vi "Shallow Search Priv.vi"(0 "Tree Dictionary In":variant, 5 "Unique ID":string, 7 "Name":string, 11 "error in":errorcluster) -> (4 "Tree Dictionary Out":variant, 6 "IDs":string[](array[string]), 15 "error out":errorcluster)   [LabVIEW 2016, in "Tree Manager.lvclass"]
uses:
  Tree Manager.lvclass
  Typedefs/Tree.ctl
  <vilib>/Utility/error.llb/Error Cluster From Error Code.vi
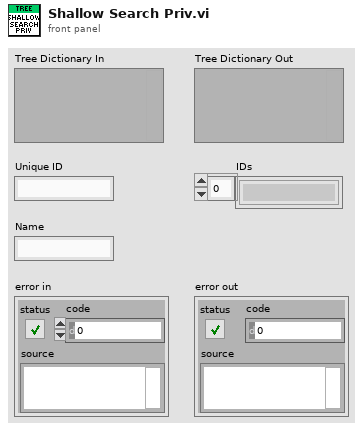
[diagram p1: front panel]
types:
  T1 = typedef "Tree Manager.lvclass/Tree.ctl" = cluster{"Unique ID":string, "Parent ID":string, "Child IDs":string[], "Data":variant, "Name":string}
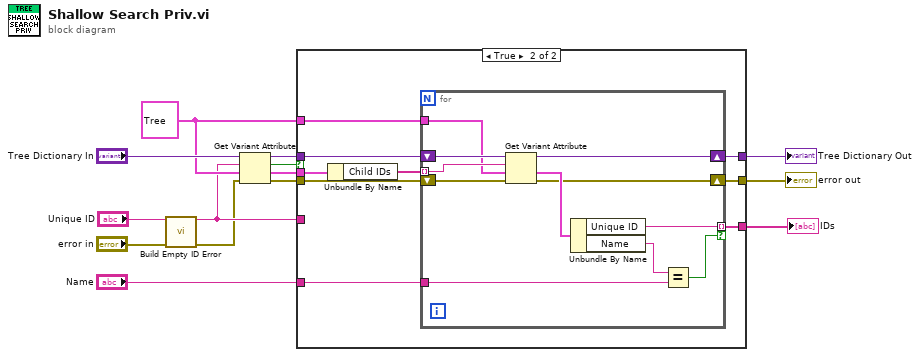
[diagram p0: block diagram]
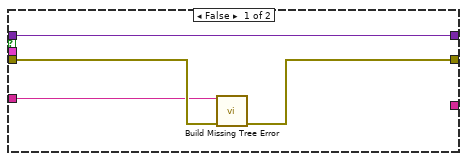
[diagram p2: hidden frame]
diagram:
  w5 = T1 {"Unique ID"="", "Parent ID"="", "Child IDs"=[], "Data"=variant, "Name"=""} ("Cluster of class private data")
  n1 = call "Build Empty ID Error.vi"("Unique ID"="Unique ID", "Error In"="error in") -> ("Unique ID Out"=w3:string, "Error Out"=w1:errorcluster)  [unwired: 12 in]
  n2 = Get Variant Attribute(Variant="Tree Dictionary In", name=w3, default value (empty Variant)=w5, error in=w1) -> (duplicate Variant=w8:variant, found=w6:bool, value=w7:T1, error out=w9:errorcluster)
  n3 = case shown="True" w6 {
    tunnel: w7 -> [_ w27]
    tunnel: w8 -> [w18 w26]
    tunnel: w9 -> [w17 w23]
    tunnel: [w15 w22] -> w12
    tunnel: [w18 w21] -> w11
    tunnel: w3 -> [w16 _]
    tunnel: "Name" -> [_ w24]
    tunnel: [_ w20] -> w13
    tunnel: w5 -> [_ w19]
    frame False {
      n4 = call "Build Missing Tree Error.vi"("Unique ID"=w16, "Error In"=w17) -> ("Error Out"=w15:errorcluster)  [unwired: 13 in]
    }
    frame True {
      n5 = Unbundle By Name(w27) -> ("Child IDs"=w25:string[])
      n6 = for {
        tunnel: w25 -> [w37] mode=indexing
        tunnel: w24 -> [w35]
        shift-right: [w31] -> w21
        shift-left: w26 -> [w38]
        tunnel: [w30] -> w20 mode=indexing if=w29
        shift-right: [w32] -> w22
        shift-left: w23 -> [w33]
        tunnel: w19 -> [w28]
        n7 = Get Variant Attribute(Variant=w38, name=w37, default value (empty Variant)=w28, error in=w33) -> (duplicate Variant=w31:variant, value=w36:T1, error out=w32:errorcluster)  [unwired: 1 out]
        n8 = Unbundle By Name(w36) -> ("Unique ID"=w30:string, "Name"=w34:string)
        n9 = Equal?(x=w34, y=w35) -> (x = y?=w29:bool)
      }
    }
  }
  "IDs" <- w13
  "error out" <- w12
  "Tree Dictionary Out" <- w11
